vi "climber_periodic.vi"(5 "Disable climberR":bool, 6 "Climber Manual Power":dbl=0.25, 7 "Disable climberL":bool, 8 "Zero Encoders":bool, 9 "Climber Down":bool, 10 "Climber Up":bool, 11 "Climber Manual Override?":bool) -> (2 "R":i32, 3 "L":i32)   [LabVIEW 2020]
uses:
  <vilib>/Rock Robotics/WPI/ThirdParty/Phoenix-LabVIEW/Motor Controller/Controls/CTRE_Phoenix_MotorControl_ControlMode.ctl
  <vilib>/Rock Robotics/WPI/ThirdParty/Phoenix-LabVIEW/Motor Controller/Get/CTRE_Phoenix_MotorController_GetSelectedSensorData.vi
  TitanLib/Lib/Piston Hold.vi
  <vilib>/Rock Robotics/WPI/Solenoid/WPI_SolenoidSetEnum.vi
  TitanLib/Lib/TitanLib.lvlib
panel:
  in  "Climber Down Pos":dbl=0.5
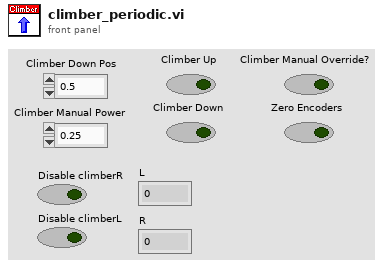
[diagram p1: front panel]
types:
  T1 = typedef "WPI_MotorControlDeviceRef.ctl" = cluster{"DeviceStatus":errorcluster, "Type":T2, "PWM":cluster{"PWM Channel":T3, "DeadBand":T4}, "CAN":cluster{"Device Number":u8, "SetOutput VI Ref":variant, "GetOutput VI Ref":variant, "Enable VI Ref":variant, "Disable VI Ref":variant, "Data":variant}, "Invert":bool, "DIO PWM":cluster{"PWM \"Enable\" Channel":T3, "DIOChannel":T5, "PWM Rate":dbl}}
  T2 = typedef "WPI_MotorControlType.ctl" = enum16{"PWM", "CAN", "DIO PWM"}
  T3 = typedef "FPGA_DIOPWMChannel.ctl" = enum8{"PWM 0", "PWM 1", "PWM 2", "PWM 3", "PWM 4", "PWM 5", "PWM 6", "PWM 7", "PWM 8", "PWM 9", "PWM MXP 0", "PWM MXP 1", "PWM MXP 2", "PWM MXP 3", "PWM MXP 4", "PWM MXP 5", "PWM MXP 6", "PWM MXP 7", "PWM MXP 8", "PWM MXP 9", "Invalid"}
  T4 = typedef "WPI_PWMDeadband.ctl" = cluster{"Name":string, "maxPositivePwm":i32, "minPositivePwm":i32, "centerPwm":i32, "maxNegativePwm":i32, "minNegativePwm":i32, "angularRange":u16}
  T5 = typedef "FPGA_DIOChannel.ctl" = enum8{"DIO 0", "DIO 1", "DIO 2", "DIO 3", "DIO 4", "DIO 5", "DIO 6", "DIO 7", "DIO 8", "DIO 9", "DIO MXP 0", "DIO MXP 1", "DIO MXP 2", "DIO MXP 3", "DIO MXP 4", "DIO MXP 5", "DIO MXP 6", "DIO MXP 7", "DIO MXP 8", "DIO MXP 9", "DIO MXP 10", "DIO MXP 11", "DIO MXP 12", "DIO MXP 13", "DIO MXP 14", "DIO MXP 15", "SPI Port CS1", "SPI Port CS2", "SPI Port CS3", "SPI Port MISO", "SPI Port MOSI", "Invalid"}
  T6 = typedef "CTRE_Phoenix_MotorControl_ControlMode.ctl" = u16
  T7 = typedef "WPI_SolenoidValue.ctl" = enum16{"Off", "On", "Forward", "Reverse"}
  T8 = typedef "WPI_SolenoidDevRef.ctl" = cluster{"DevStatus":errorcluster, "Pneumatics Control Module":u8, "Forward Solenoid Channel":T9, "Reverse Solenoid Channel":T9}
  T9 = typedef "WPI_SolenoidChannel.ctl" = enum8{"Solenoid 0", "Solenoid 1", "Solenoid 2", "Solenoid 3", "Solenoid 4", "Solenoid 5", "Solenoid 6", "Solenoid 7", "Solenoid 8", "Solenoid 9", "Solenoid 10", "Solenoid 11", "Solenoid 12", "Solenoid 13", "Solenoid 14", "Solenoid 15", "Invalid"}
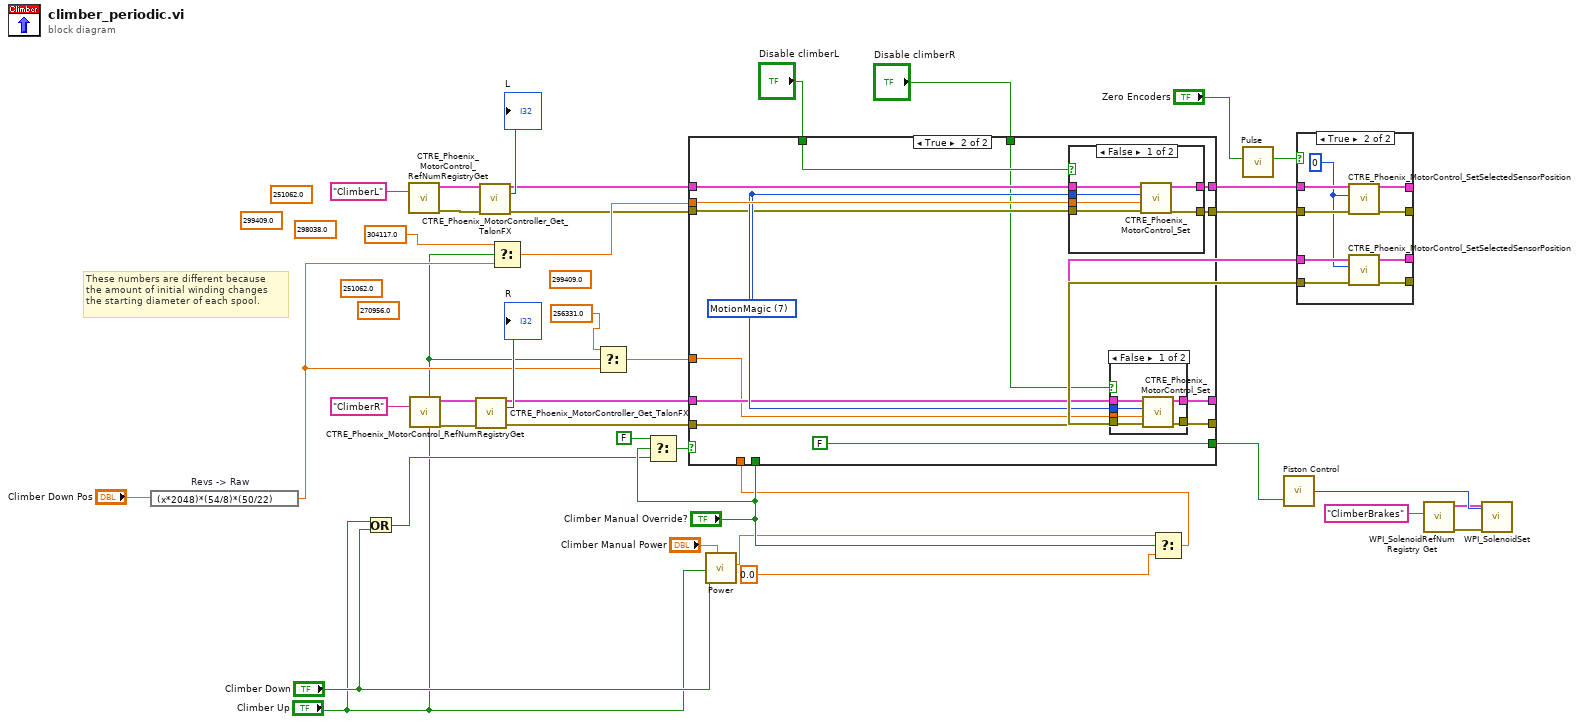
[diagram p0: block diagram]
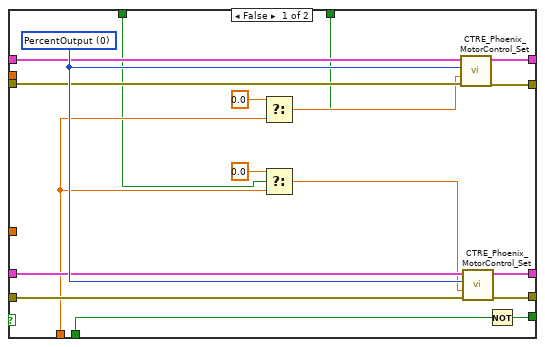
[diagram p3: hidden frame]
diagram:
  (unwired) 251062.0 ("t")
  (unwired) 299409.0 ("t")
  (unwired) 270956.0 ("t")
  (unwired) 298038.0 ("t")
  (unwired) 251062.0 ("t")
  (unwired) 299409.0 ("t")
  # "These numbers are different because\nthe amount of initial winding changes\nthe starting diameter of each spool."
  n1 = expression code="(x*2048)*(54/8)*(50/22)" "Revs -> Raw"("Climber Down Pos") -> (w5:dbl)
  n2 = Or(x="Climber Up", y="Climber Down") -> (x .or. y?=w32:bool)
  n3 = call <vilib>:"CTRE_Phoenix_MotorControl_RefNumRegistryGet.vi"("refnum name"="ClimberL") -> ("error out"=w16:errorcluster, "PhoenixMotorControlDevRef"=w17:T1)  [unwired: 9 in]
  n4 = call <vilib>:"CTRE_Phoenix_MotorControl_RefNumRegistryGet.vi"("refnum name"="ClimberR") -> ("error out"=w14:errorcluster, "PhoenixMotorControlDevRef"=w15:T1)  [unwired: 9 in]
  n5 = call-poly <vilib>:"CTRE_Phoenix_MotorController_Get_TalonFX.vi"("PhoenixMotorControlDevRef"=w15, "error in"=w14) -> ("PhoenixMotorControlDevRef"=w11:T1, "Position (Raw Sensor Units)"=→"R":i32, "error out"=w10:errorcluster)  [unwired: 10 in, 1 out]
  n6 = call-poly <vilib>:"CTRE_Phoenix_MotorController_Get_TalonFX.vi"("PhoenixMotorControlDevRef"=w17, "error in"=w16) -> ("PhoenixMotorControlDevRef"=w8:T1, "Position (Raw Sensor Units)"=→"L":i32, "error out"=w9:errorcluster)  [unwired: 10 in, 1 out]
  n7 = Select(t=304117.0, s="Climber Up", f=w5) -> (s? t:f=w27:dbl)
  n8 = Select(t=256331.0, s="Climber Up", f=w5) -> (s? t:f=w7:dbl)
  n9 = Select(t=FALSE, s="Climber Manual Override?", f=w32) -> (s? t:f=w31:bool)
  n10 = call "Power.vi"("Positive Power"="Climber Manual Power", "Negative"="Climber Down", "Positive"="Climber Up") -> ("Output"=w28:dbl)  [unwired: 8 in]
  n11 = Select(t=w28, s="Climber Manual Override?", f=0.0 ("Output")) -> (s? t:f=w30:dbl)
  n12 = case shown="True" w31 {
    tunnel: w27 -> [_ w73]
    tunnel: w8 -> [w58 w71]
    tunnel: w11 -> [w56 w70]
    tunnel: w10 -> [w55 w69]
    tunnel: w9 -> [w57 w68]
    tunnel: w30 -> [w48 _]
    tunnel: [w54 w67] -> w21
    tunnel: [w53 w66] -> w22
    tunnel: [w52 w65] -> w23
    tunnel: [w51 w64] -> w24
    tunnel: [w50 FALSE ("t")] -> w38
    tunnel: "Climber Manual Override?" -> [w49 _]
    tunnel: "Disable climberR" -> [w43 w61]
    tunnel: "Disable climberL" -> [w42 w62]
    tunnel: w7 -> [_ w60]
    frame False {
      w59 = T6 0 items=["PercentOutput"=0, "Position"=1, "Velocity"=2, "Current"=3, "Follower"=5, "MotionProfile"=6, "MotionMagic"=7, "MotionProfileArc"=10, "Disabled"=15] ("Control Mode")
      n13 = Select(t=0.0, s=w43, f=w48) -> (s? t:f=w46:dbl)
      n14 = Select(t=0.0, s=w42, f=w48) -> (s? t:f=w47:dbl)
      n15 = call <vilib>:"CTRE_Phoenix_MotorControl_Set.vi"("error in (no error)"=w57, "Output"=w46, "Control Mode"=w59, "PhoenixMotorControlDevRef"=w58) -> ("error out"=w53:errorcluster, "PhoenixMotorControlDevRef"=w54:T1)  [unwired: 6 in]
      n16 = call <vilib>:"CTRE_Phoenix_MotorControl_Set.vi"("error in (no error)"=w55, "Output"=w47, "Control Mode"=w59, "PhoenixMotorControlDevRef"=w56) -> ("error out"=w51:errorcluster, "PhoenixMotorControlDevRef"=w52:T1)  [unwired: 6 in]
      n17 = Not(x=w49) -> (.not. x?=w50:bool)
    }
    frame True {
      w72 = T6 7 items=["PercentOutput"=0, "Position"=1, "Velocity"=2, "Current"=3, "Follower"=5, "MotionProfile"=6, "MotionMagic"=7, "MotionProfileArc"=10, "Disabled"=15] ("Control Mode")
      n18 = case shown="False" w62 {
        tunnel: w73 -> [w87 _]
        tunnel: w72 -> [w86 _]
        tunnel: w71 -> [w85 w89]
        tunnel: w68 -> [w84 w88]
        tunnel: [w83 w89] -> w67
        tunnel: [w82 w88] -> w66
        frame False {
          n19 = call <vilib>:"CTRE_Phoenix_MotorControl_Set.vi"("error in (no error)"=w84, "Output"=w87, "Control Mode"=w86, "PhoenixMotorControlDevRef"=w85) -> ("error out"=w82:errorcluster, "PhoenixMotorControlDevRef"=w83:T1)  [unwired: 6 in]
        }
        frame True {
        }
      }
      n20 = case shown="False" w61 {
        tunnel: w60 -> [w79 _]
        tunnel: w72 -> [w78 _]
        tunnel: w70 -> [w77 w81]
        tunnel: w69 -> [w76 w80]
        tunnel: [w75 w81] -> w65
        tunnel: [w74 w80] -> w64
        frame False {
          n21 = call <vilib>:"CTRE_Phoenix_MotorControl_Set.vi"("error in (no error)"=w76, "Output"=w79, "Control Mode"=w78, "PhoenixMotorControlDevRef"=w77) -> ("error out"=w74:errorcluster, "PhoenixMotorControlDevRef"=w75:T1)  [unwired: 6 in]
        }
        frame True {
        }
      }
    }
  }
  n22 = call "Pulse.vi"("Input"="Zero Encoders") -> ("Output"=w25:bool)  [unwired: 10 in]
  n23 = call-poly "Piston Control.vi"("Input"=w38) -> ("Output"=w37:T7)  [unwired: 1 in]
  n24 = case shown="True" w25 {
    tunnel: w21 -> [w93 w102]
    tunnel: w22 -> [w92 w101]
    tunnel: w23 -> [w91 w100]
    tunnel: w24 -> [w90 w99]
    tunnel: [w93 w97] -> _
    tunnel: [w92 w96] -> _
    tunnel: [w91 w95] -> _
    tunnel: [w90 w94] -> _
    frame False {
    }
    frame True {
      w98 = 0 ("New Sensor Position")
      n25 = call <vilib>:"CTRE_Phoenix_MotorControl_SetSelectedSensorPosition.vi"("error in (no error)"=w101, "New Sensor Position"=w98, "PhoenixMotorControlDevRef"=w102) -> ("error out"=w96:errorcluster, "PhoenixMotorControlDevRef"=w97:T1)  [unwired: 7 in]
      n26 = call <vilib>:"CTRE_Phoenix_MotorControl_SetSelectedSensorPosition.vi"("error in (no error)"=w99, "New Sensor Position"=w98, "PhoenixMotorControlDevRef"=w100) -> ("error out"=w94:errorcluster, "PhoenixMotorControlDevRef"=w95:T1)  [unwired: 7 in]
    }
  }
  n27 = call <vilib>:"WPI_SolenoidRefNum Registry Get.vi"("refnum name"="ClimberBrakes") -> ("error out"=w35:errorcluster, "SolenoidDevRef"=w34:T8)  [unwired: 9 in]
  n28 = call-poly <vilib>:"WPI_SolenoidSet.vi"("error in (no error)"=w35, "Value"=w37, "SolenoidDevRef"=w34) -> ()  [unwired: 7 in, 2 out]
